vi "RTS Check WH Reset.vi"(8 "Error In":errorcluster, 10 "TDMS Data Save in":T4, 11 "Device Connections in":T1 {"MX5"."Channel Number (1)" min=1 max=60 step=1; "MX5"."FIFO Number (0)" min=-1 max=2 step=1; "MX4"."Channel Number (1)" min=1 max=60 step=1; "MX4"."FIFO Number (0)" min=-1 max=2 step=1; "MX3"."Channel Number (1)" min=1 max=60 step=1; "MX3"."FIFO Number (0)" min=-1 max=2 step=1; "MX2"."Channel Number (1)" min=1 max=60 step=1; "MX2"."FIFO Number (0)" min=-1 max=2 step=1; "MX1"."Channel Number (1)" min=1 max=60 step=1; "MX1"."FIFO Number (0)" min=-1 max=2 step=1}) -> (0 "Error Out":errorcluster, 3 "Device Connections out":T1={"Wago ModBus Connection"=refnum, "APLUS 1 Modbus Connection"=refnum, "APLUS 2 Modbus Connection"=refnum, "APLUS 3 Modbus Connection"=refnum, "APLUS 4 Modbus Connection"=refnum, "APLUS 5 Modbus Connection"=refnum, "APLUS 6 Modbus Connection"=refnum, "APLUS 7 Modbus Connection"=refnum, "APLUS 8 Modbus Connection"=refnum, "MX 1 VISA Connection"="", "MX 2 VISA Connection"="", "MX 3 VISA Connection"="", "MX 4 VISA Connection"="", "MX 5 VISA Connection"="", "MX1"={"Base Time"=0, "Session Number"=0, "Last Data Number"={"High"=-1, "Low"=4294967295}, "Channel List"=[], "FIFO Number (0)"=0, "Channel Number (1)"=1, "Select FIFO or Channel (F:Channel)"=FALSE, "MX100 Data"={"Measurement Values out"=[], "Date/Time"=""}}, "MX2"={"Base Time"=0, "Session Number"=0, "Last Data Number"={"High"=-1, "Low"=4294967295}, "Channel List"=[], "FIFO Number (0)"=0, "Channel Number (1)"=1, "Select FIFO or Channel (F:Channel)"=FALSE, "MX100 Data"={"Measurement Values out"=[], "Date/Time"=""}}, "MX3"={"Base Time"=0, "Session Number"=0, "Last Data Number"={"High"=-1, "Low"=4294967295}, "Channel List"=[], "FIFO Number (0)"=0, "Channel Number (1)"=1, "Select FIFO or Channel (F:Channel)"=FALSE, "MX100 Data"={"Measurement Values out"=[], "Date/Time"=""}}, "MX4"={"Base Time"=0, "Session Number"=0, "Last Data Number"={"High"=-1, "Low"=4294967295}, "Channel List"=[], "FIFO Number (0)"=0, "Channel Number (1)"=1, "Select FIFO or Channel (F:Channel)"=FALSE, "MX100 Data"={"Measurement Values out"=[], "Date/Time"=""}}, "MX5"={"Base Time"=0, "Session Number"=0, "Last Data Number"={"High"=-1, "Low"=4294967295}, "Channel List"=[], "FIFO Number (0)"=0, "Channel Number (1)"=1, "Select FIFO or Channel (F:Channel)"=FALSE, "MX100 Data"={"Measurement Values out"=[], "Date/Time"=""}}} {"MX5"."Channel Number (1)" min=1 max=60 step=1; "MX5"."FIFO Number (0)" min=-1 max=2 step=1; "MX4"."Channel Number (1)" min=1 max=60 step=1; "MX4"."FIFO Number (0)" min=-1 max=2 step=1; "MX3"."Channel Number (1)" min=1 max=60 step=1; "MX3"."FIFO Number (0)" min=-1 max=2 step=1; "MX2"."Channel Number (1)" min=1 max=60 step=1; "MX2"."FIFO Number (0)" min=-1 max=2 step=1; "MX1"."Channel Number (1)" min=1 max=60 step=1; "MX1"."FIFO Number (0)" min=-1 max=2 step=1})   [LabVIEW 2016]
uses:
  Type Definitions/RTS Modbus Connections.ctl
  <vilib>/NI/Modbus Library/API/Master/Modbus Master.lvclass
  Drivers/Yokogawa MX100/Type Definitions/MX100 Initialization.ctl
  Drivers/Yokogawa MX100/Type Definitions/MX100 Data.ctl
  Type Definitions/RTS TDMS Filename Locations.ctl
  Type Definitions/RTS Save References.ctl
  Utility/Save File/Save File.lvlib
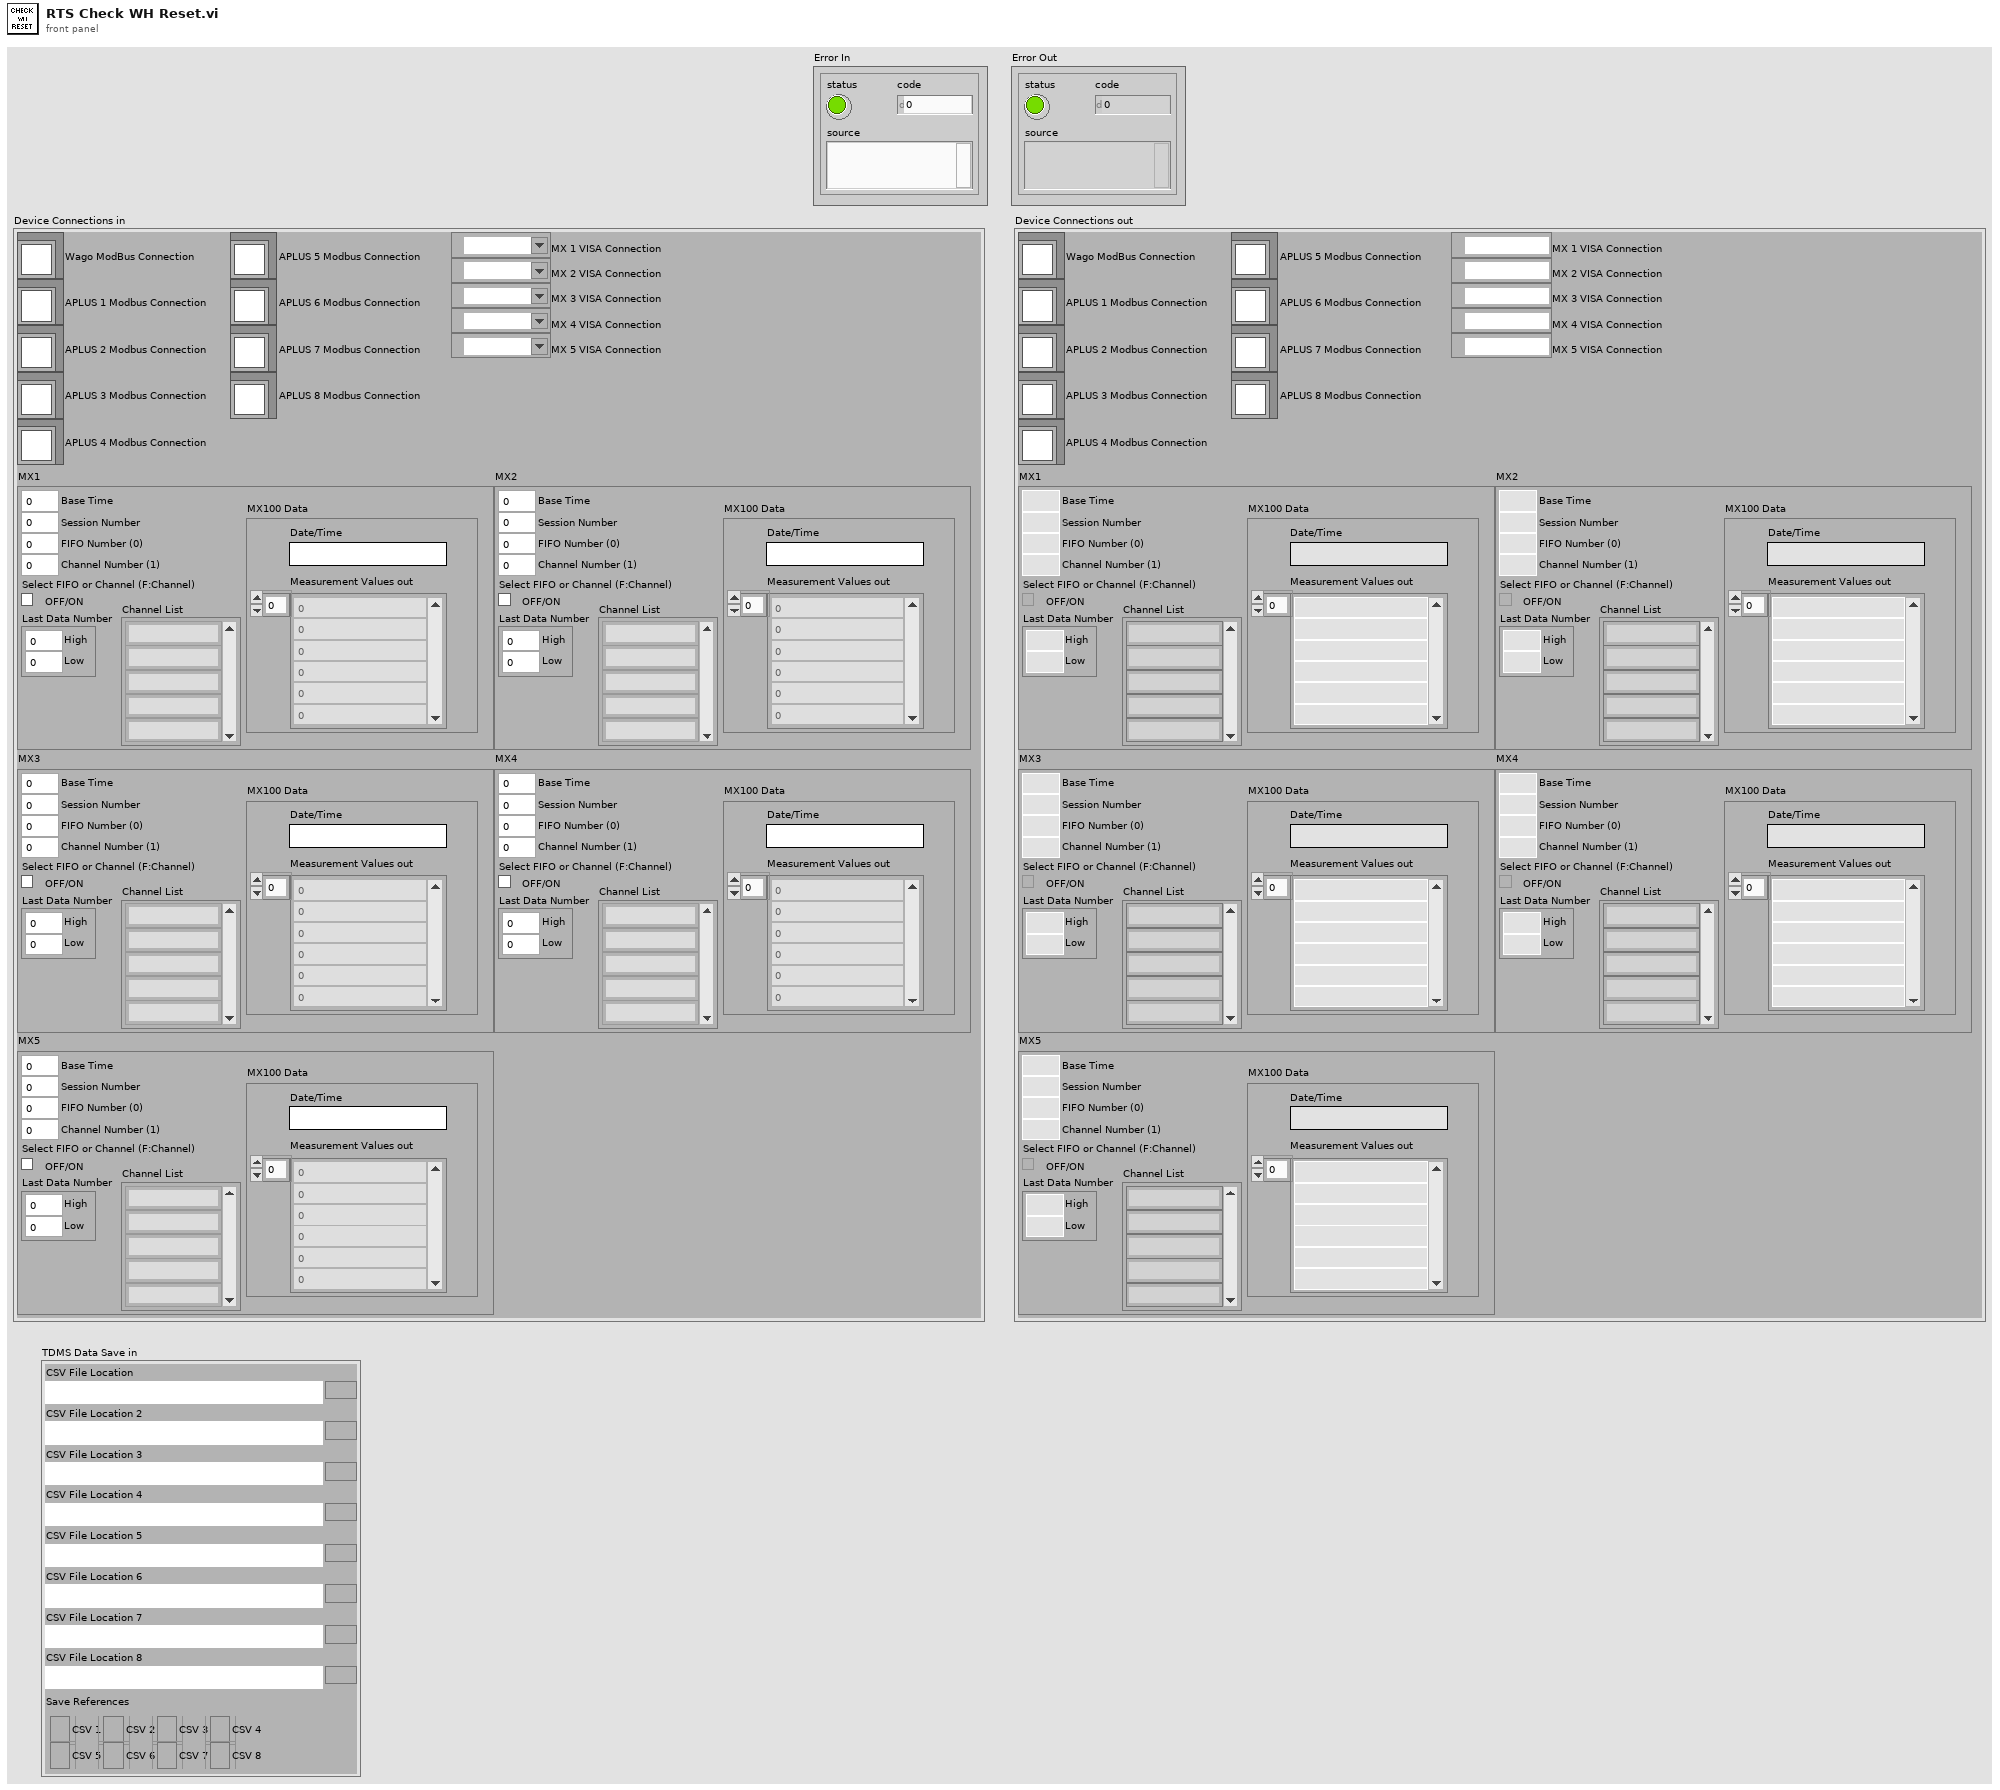
[diagram p1: front panel]
types:
  T1 = typedef "RTS Modbus Connections.ctl" = cluster{"Wago ModBus Connection":refnum<class "Modbus Master.lvclass">, "APLUS 1 Modbus Connection":refnum<class "Modbus Master.lvclass">, "APLUS 2 Modbus Connection":refnum<class "Modbus Master.lvclass">, "APLUS 3 Modbus Connection":refnum<class "Modbus Master.lvclass">, "APLUS 4 Modbus Connection":refnum<class "Modbus Master.lvclass">, "APLUS 5 Modbus Connection":refnum<class "Modbus Master.lvclass">, "APLUS 6 Modbus Connection":refnum<class "Modbus Master.lvclass">, "APLUS 7 Modbus Connection":refnum<class "Modbus Master.lvclass">, "APLUS 8 Modbus Connection":refnum<class "Modbus Master.lvclass">, "MX 1 VISA Connection":refnum<visa-resource-name>, "MX 2 VISA Connection":refnum<visa-resource-name>, "MX 3 VISA Connection":refnum<visa-resource-name>, "MX 4 VISA Connection":refnum<visa-resource-name>, "MX 5 VISA Connection":refnum<visa-resource-name>, "MX1":T2, "MX2":T2, "MX3":T2, "MX4":T2, "MX5":T2}
  T2 = typedef "MX100 Initialization.ctl" = cluster{"Base Time":i32, "Session Number":i32, "Last Data Number":cluster{"High":i32, "Low":u32}, "Channel List":string[], "FIFO Number (0)":i32, "Channel Number (1)":i32, "Select FIFO or Channel (F:Channel)":bool, "MX100 Data":T3}
  T3 = typedef "MX100 Data.ctl" = cluster{"Measurement Values out":dbl[], "Date/Time":string}
  T4 = typedef "RTS TDMS Filename Locations.ctl" = cluster{"CSV File Location":path, "CSV File Location 2":path, "CSV File Location 3":path, "CSV File Location 4":path, "CSV File Location 5":path, "CSV File Location 6":path, "CSV File Location 7":path, "CSV File Location 8":path, "Save References":T5}
  T5 = typedef "RTS Save References.ctl" = cluster{"CSV 1":refnum<file>, "CSV 2":refnum<file>, "CSV 3":refnum<file>, "CSV 4":refnum<file>, "CSV 5":refnum<file>, "CSV 6":refnum<file>, "CSV 7":refnum<file>, "CSV 8":refnum<file>}
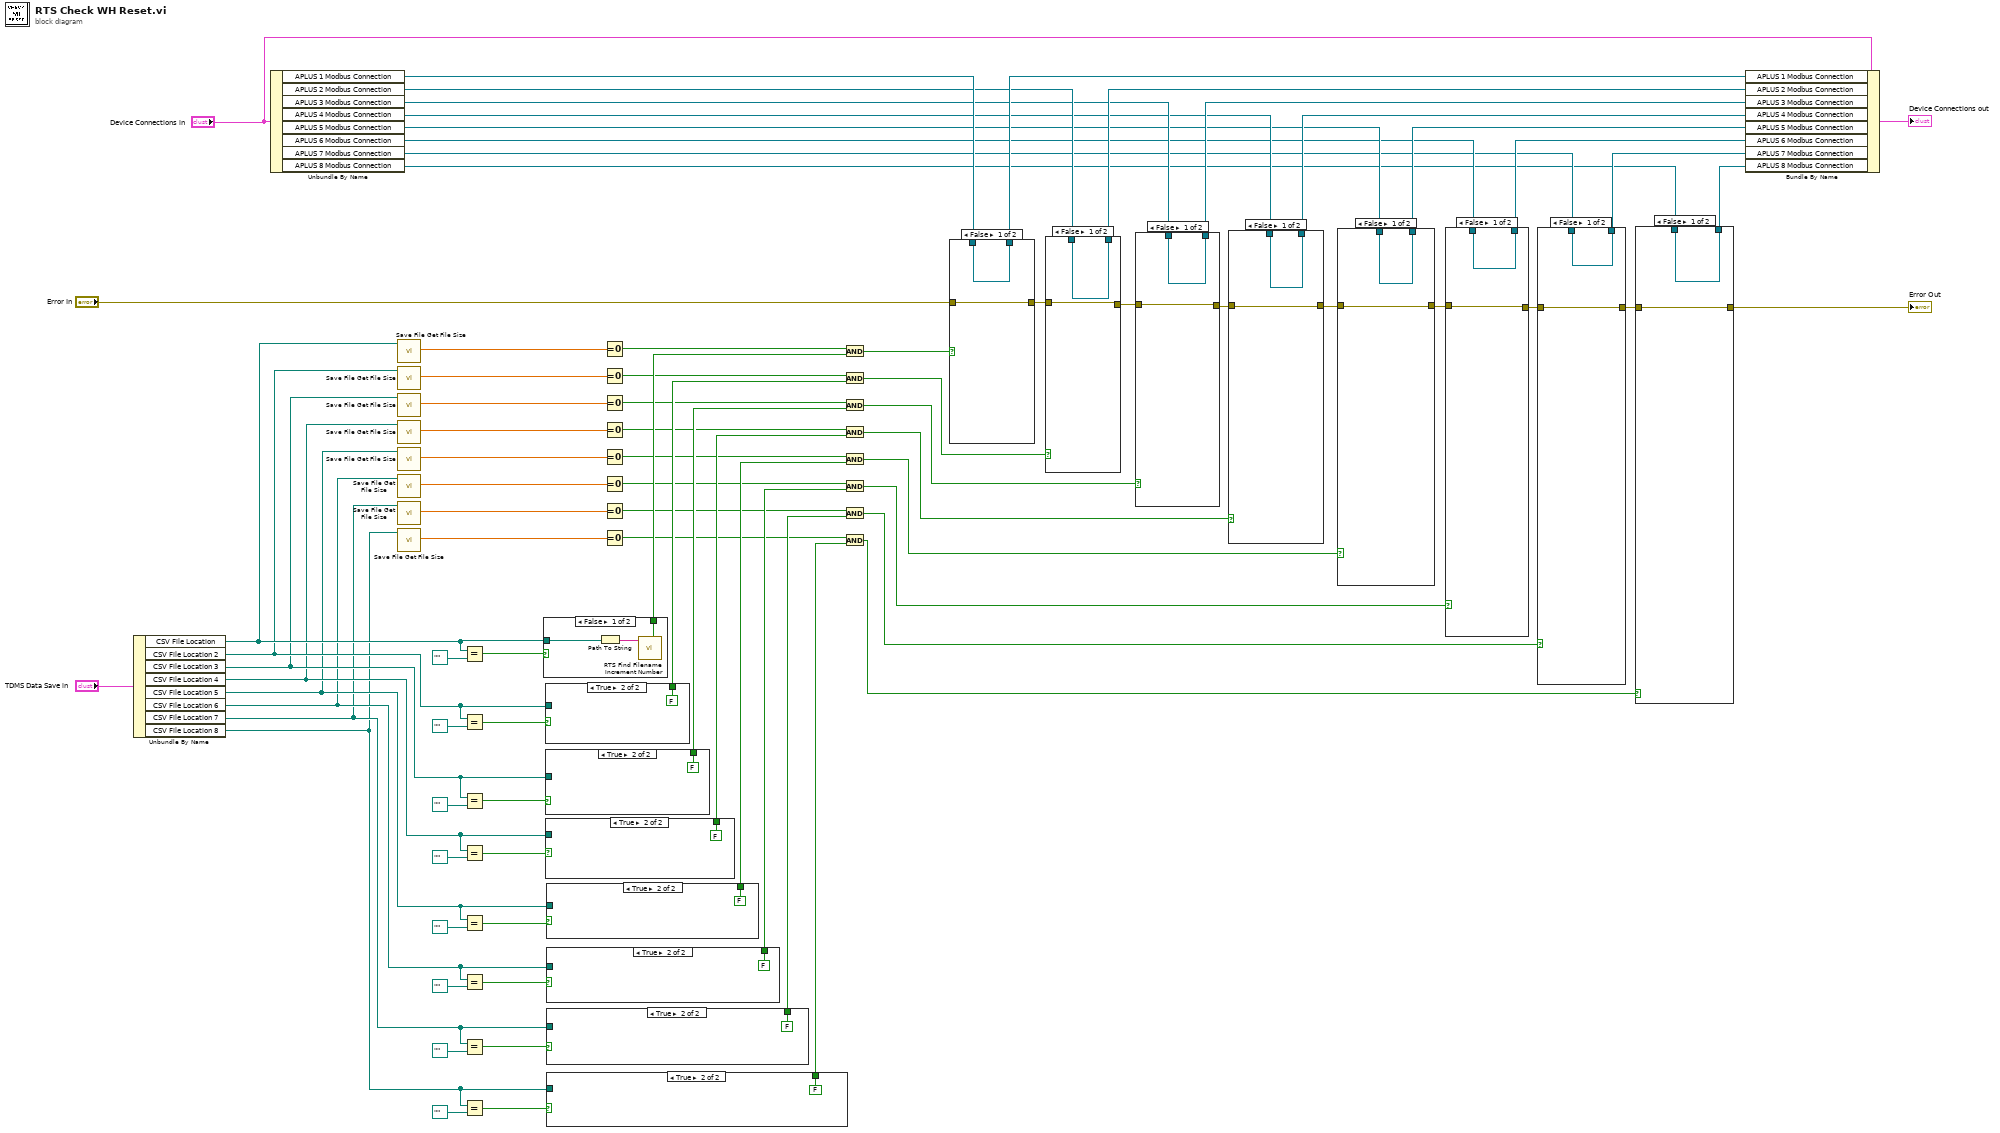
[diagram p0: block diagram]
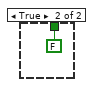
[diagram p2: hidden frame]
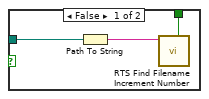
[diagram p3: hidden frame]
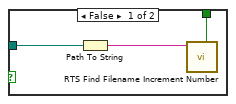
[diagram p4: hidden frame]
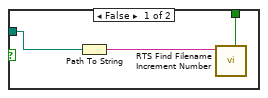
[diagram p5: hidden frame]
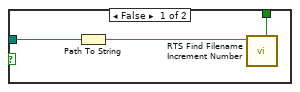
[diagram p6: hidden frame]
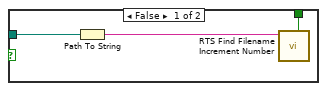
[diagram p7: hidden frame]
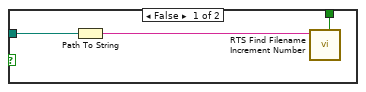
[diagram p8: hidden frame]
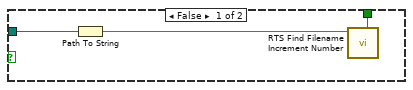
[diagram p9: hidden frame]
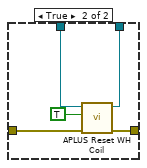
[diagram p10: hidden frame]
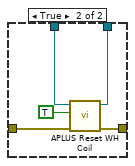
[diagram p11: hidden frame]
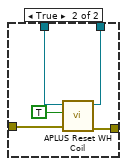
[diagram p12: hidden frame]
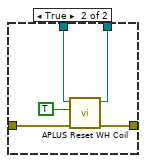
[diagram p13: hidden frame]
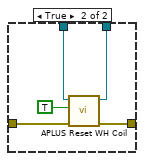
[diagram p14: hidden frame]
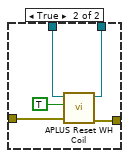
[diagram p15: hidden frame]
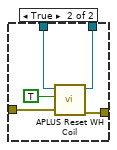
[diagram p16: hidden frame]
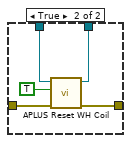
[diagram p17: hidden frame]
diagram:
  n1 = Unbundle By Name("TDMS Data Save in") -> ("CSV File Location"=w16:path, "CSV File Location 2"=w14:path, "CSV File Location 3"=w12:path, "CSV File Location 4"=w10:path, "CSV File Location 5"=w8:path, "CSV File Location 6"=w6:path, "CSV File Location 7"=w4:path, "CSV File Location 8"=w2:path)
  n2 = Unbundle By Name("Device Connections in") -> ("APLUS 1 Modbus Connection"=w73:refnum<class "Modbus Master.lvclass">, "APLUS 2 Modbus Connection"=w71:refnum<class "Modbus Master.lvclass">, "APLUS 3 Modbus Connection"=w69:refnum<class "Modbus Master.lvclass">, "APLUS 4 Modbus Connection"=w67:refnum<class "Modbus Master.lvclass">, "APLUS 5 Modbus Connection"=w65:refnum<class "Modbus Master.lvclass">, "APLUS 6 Modbus Connection"=w63:refnum<class "Modbus Master.lvclass">, "APLUS 7 Modbus Connection"=w61:refnum<class "Modbus Master.lvclass">, "APLUS 8 Modbus Connection"=w59:refnum<class "Modbus Master.lvclass">)
  n3 = call "Save File Get File Size.vi"("Old path"=w16) -> ("File Size MB"=w15:dbl)  [unwired: 8 in, 2 out]
  n4 = call "Save File Get File Size.vi"("Old path"=w14) -> ("File Size MB"=w13:dbl)  [unwired: 8 in, 2 out]
  n5 = call "Save File Get File Size.vi"("Old path"=w12) -> ("File Size MB"=w11:dbl)  [unwired: 8 in, 2 out]
  n6 = call "Save File Get File Size.vi"("Old path"=w10) -> ("File Size MB"=w9:dbl)  [unwired: 8 in, 2 out]
  n7 = call "Save File Get File Size.vi"("Old path"=w8) -> ("File Size MB"=w7:dbl)  [unwired: 8 in, 2 out]
  n8 = call "Save File Get File Size.vi"("Old path"=w6) -> ("File Size MB"=w5:dbl)  [unwired: 8 in, 2 out]
  n9 = call "Save File Get File Size.vi"("Old path"=w4) -> ("File Size MB"=w3:dbl)  [unwired: 8 in, 2 out]
  n10 = call "Save File Get File Size.vi"("Old path"=w2) -> ("File Size MB"=w1:dbl)  [unwired: 8 in, 2 out]
  n11 = Equal?(x=w16, y=path "") -> (x = y?=w17:bool)
  n12 = Equal?(x=w14, y=path "") -> (x = y?=w19:bool)
  n13 = Equal?(x=w12, y=path "") -> (x = y?=w21:bool)
  n14 = Equal?(x=w10, y=path "") -> (x = y?=w23:bool)
  n15 = Equal?(x=w8, y=path "") -> (x = y?=w25:bool)
  n16 = Equal?(x=w6, y=path "") -> (x = y?=w27:bool)
  n17 = Equal?(x=w4, y=path "") -> (x = y?=w29:bool)
  n18 = Equal?(x=w2, y=path "") -> (x = y?=w31:bool)
  n19 = case shown="False" w17 {
    tunnel: w16 -> [w87 _]
    tunnel: [w85 FALSE ("No Match")] -> w55
    frame False {
      n20 = Path To String(path=w87) -> (string=w86:string)
      n21 = call "RTS Find Filename Increment Number.vi"("Input name in"=w86) -> ("No Match"=w85:bool)  [unwired: 7 in, 3 out]
    }
    frame True {
    }
  }
  n22 = case shown="True" w19 {
    tunnel: w14 -> [w90 _]
    tunnel: [w89 FALSE ("No Match")] -> w52
    frame False {
      n23 = Path To String(path=w90) -> (string=w91:string)
      n24 = call "RTS Find Filename Increment Number.vi"("Input name in"=w91) -> ("No Match"=w89:bool)  [unwired: 7 in, 3 out]
    }
    frame True {
    }
  }
  n25 = case shown="True" w21 {
    tunnel: w12 -> [w94 _]
    tunnel: [w93 FALSE ("No Match")] -> w49
    frame False {
      n26 = Path To String(path=w94) -> (string=w95:string)
      n27 = call "RTS Find Filename Increment Number.vi"("Input name in"=w95) -> ("No Match"=w93:bool)  [unwired: 7 in, 3 out]
    }
    frame True {
    }
  }
  n28 = case shown="True" w23 {
    tunnel: w10 -> [w98 _]
    tunnel: [w97 FALSE ("No Match")] -> w45
    frame False {
      n29 = Path To String(path=w98) -> (string=w99:string)
      n30 = call "RTS Find Filename Increment Number.vi"("Input name in"=w99) -> ("No Match"=w97:bool)  [unwired: 7 in, 3 out]
    }
    frame True {
    }
  }
  n31 = case shown="True" w25 {
    tunnel: w8 -> [w102 _]
    tunnel: [w101 FALSE ("No Match")] -> w42
    frame False {
      n32 = Path To String(path=w102) -> (string=w103:string)
      n33 = call "RTS Find Filename Increment Number.vi"("Input name in"=w103) -> ("No Match"=w101:bool)  [unwired: 7 in, 3 out]
    }
    frame True {
    }
  }
  n34 = case shown="True" w27 {
    tunnel: w6 -> [w106 _]
    tunnel: [w105 FALSE ("No Match")] -> w39
    frame False {
      n35 = Path To String(path=w106) -> (string=w107:string)
      n36 = call "RTS Find Filename Increment Number.vi"("Input name in"=w107) -> ("No Match"=w105:bool)  [unwired: 7 in, 3 out]
    }
    frame True {
    }
  }
  n37 = case shown="True" w29 {
    tunnel: w4 -> [w110 _]
    tunnel: [w109 FALSE ("No Match")] -> w36
    frame False {
      n38 = Path To String(path=w110) -> (string=w111:string)
      n39 = call "RTS Find Filename Increment Number.vi"("Input name in"=w111) -> ("No Match"=w109:bool)  [unwired: 7 in, 3 out]
    }
    frame True {
    }
  }
  n40 = case shown="True" w31 {
    tunnel: w2 -> [w114 _]
    tunnel: [w113 FALSE ("No Match")] -> w33
    frame False {
      n41 = Path To String(path=w114) -> (string=w115:string)
      n42 = call "RTS Find Filename Increment Number.vi"("Input name in"=w115) -> ("No Match"=w113:bool)  [unwired: 7 in, 3 out]
    }
    frame True {
    }
  }
  n43 = Equal To 0?(x=w15) -> (x = 0?=w56:bool)
  n44 = Equal To 0?(x=w13) -> (x = 0?=w53:bool)
  n45 = Equal To 0?(x=w11) -> (x = 0?=w50:bool)
  n46 = Equal To 0?(x=w9) -> (x = 0?=w47:bool)
  n47 = Equal To 0?(x=w7) -> (x = 0?=w44:bool)
  n48 = Equal To 0?(x=w5) -> (x = 0?=w41:bool)
  n49 = Equal To 0?(x=w3) -> (x = 0?=w38:bool)
  n50 = Equal To 0?(x=w1) -> (x = 0?=w35:bool)
  n51 = And(x=w56, y=w55) -> (x .and. y?=w54:bool)
  n52 = And(x=w53, y=w52) -> (x .and. y?=w51:bool)
  n53 = And(x=w50, y=w49) -> (x .and. y?=w48:bool)
  n54 = And(x=w47, y=w45) -> (x .and. y?=w46:bool)
  n55 = And(x=w44, y=w42) -> (x .and. y?=w43:bool)
  n56 = And(x=w41, y=w39) -> (x .and. y?=w40:bool)
  n57 = And(x=w38, y=w36) -> (x .and. y?=w37:bool)
  n58 = And(x=w35, y=w33) -> (x .and. y?=w34:bool)
  n59 = case shown="False" w54 {
    tunnel: [w117 w122] -> w82
    tunnel: "Error In" -> [w117 w121]
    tunnel: w73 -> [w118 w120]
    tunnel: [w118 w119] -> w72
    frame False {
    }
    frame True {
      n60 = call "APLUS Reset WH Coil.vi"("Error In"=w121, "Reset WattHours"=TRUE, "Modbus Master in"=w120) -> ("Error Out"=w122:errorcluster, "Modbus Master out"=w119:refnum<class "Modbus Master.lvclass">)  [unwired: 7 in]
    }
  }
  n61 = case shown="False" w51 {
    tunnel: w82 -> [w124 w129]
    tunnel: [w124 w128] -> w81
    tunnel: w71 -> [w125 w127]
    tunnel: [w125 w126] -> w70
    frame False {
    }
    frame True {
      n62 = call "APLUS Reset WH Coil.vi"("Error In"=w129, "Reset WattHours"=TRUE, "Modbus Master in"=w127) -> ("Error Out"=w128:errorcluster, "Modbus Master out"=w126:refnum<class "Modbus Master.lvclass">)  [unwired: 7 in]
    }
  }
  n63 = case shown="False" w48 {
    tunnel: w81 -> [w131 w136]
    tunnel: [w131 w135] -> w80
    tunnel: w69 -> [w132 w134]
    tunnel: [w132 w133] -> w68
    frame False {
    }
    frame True {
      n64 = call "APLUS Reset WH Coil.vi"("Error In"=w136, "Reset WattHours"=TRUE, "Modbus Master in"=w134) -> ("Error Out"=w135:errorcluster, "Modbus Master out"=w133:refnum<class "Modbus Master.lvclass">)  [unwired: 7 in]
    }
  }
  n65 = case shown="False" w46 {
    tunnel: w80 -> [w138 w143]
    tunnel: [w138 w142] -> w79
    tunnel: w67 -> [w139 w141]
    tunnel: [w139 w140] -> w66
    frame False {
    }
    frame True {
      n66 = call "APLUS Reset WH Coil.vi"("Error In"=w143, "Reset WattHours"=TRUE, "Modbus Master in"=w141) -> ("Error Out"=w142:errorcluster, "Modbus Master out"=w140:refnum<class "Modbus Master.lvclass">)  [unwired: 7 in]
    }
  }
  n67 = case shown="False" w43 {
    tunnel: w79 -> [w145 w150]
    tunnel: [w145 w149] -> w78
    tunnel: w65 -> [w146 w148]
    tunnel: [w146 w147] -> w64
    frame False {
    }
    frame True {
      n68 = call "APLUS Reset WH Coil.vi"("Error In"=w150, "Reset WattHours"=TRUE, "Modbus Master in"=w148) -> ("Error Out"=w149:errorcluster, "Modbus Master out"=w147:refnum<class "Modbus Master.lvclass">)  [unwired: 7 in]
    }
  }
  n69 = case shown="False" w40 {
    tunnel: w78 -> [w152 w157]
    tunnel: [w152 w156] -> w77
    tunnel: w63 -> [w153 w155]
    tunnel: [w153 w154] -> w62
    frame False {
    }
    frame True {
      n70 = call "APLUS Reset WH Coil.vi"("Error In"=w157, "Reset WattHours"=TRUE, "Modbus Master in"=w155) -> ("Error Out"=w156:errorcluster, "Modbus Master out"=w154:refnum<class "Modbus Master.lvclass">)  [unwired: 7 in]
    }
  }
  n71 = case shown="False" w37 {
    tunnel: w77 -> [w159 w164]
    tunnel: [w159 w163] -> w76
    tunnel: w61 -> [w160 w162]
    tunnel: [w160 w161] -> w60
    frame False {
    }
    frame True {
      n72 = call "APLUS Reset WH Coil.vi"("Error In"=w164, "Reset WattHours"=TRUE, "Modbus Master in"=w162) -> ("Error Out"=w163:errorcluster, "Modbus Master out"=w161:refnum<class "Modbus Master.lvclass">)  [unwired: 7 in]
    }
  }
  n73 = case shown="False" w34 {
    tunnel: w76 -> [w166 w171]
    tunnel: [w166 w170] -> w75
    tunnel: w59 -> [w167 w169]
    tunnel: [w167 w168] -> w58
    frame False {
    }
    frame True {
      n74 = call "APLUS Reset WH Coil.vi"("Error In"=w171, "Reset WattHours"=TRUE, "Modbus Master in"=w169) -> ("Error Out"=w170:errorcluster, "Modbus Master out"=w168:refnum<class "Modbus Master.lvclass">)  [unwired: 7 in]
    }
  }
  "Error Out" <- w75
  n75 = Bundle By Name(cluster="Device Connections in", "APLUS 1 Modbus Connection"=w72, "APLUS 2 Modbus Connection"=w70, "APLUS 3 Modbus Connection"=w68, "APLUS 4 Modbus Connection"=w66, "APLUS 5 Modbus Connection"=w64, "APLUS 6 Modbus Connection"=w62, "APLUS 7 Modbus Connection"=w60, "APLUS 8 Modbus Connection"=w58) -> (→"Device Connections out":T1)
